vi "NotchFilter.vi"(3 "Image In":T1 {"Dialogs" format="%.0b"}) -> (0 "FFT Out":T1 {"Dialogs" format="%.0b"}, 1 "Image Out":T1 {"Dialogs" format="%.0b"})   [LabVIEW 2024]
doc: "This VI removes the mean (0 freq) from the image. It only works on greyscale images."
uses:
  <userlib>/ImageProcessing/QTLIB_2595_LV86/QT_Image.ctl
panel:
  # "This VI removes the mean (0 freq) from the image.  It only works on greyscale images."
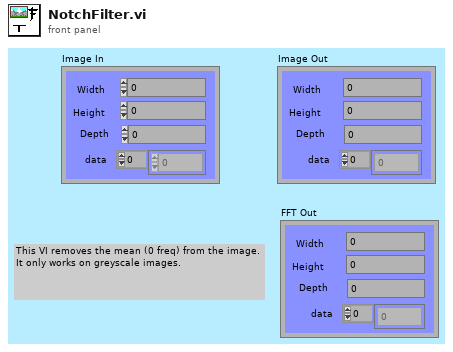
[diagram p1: front panel]
types:
  T1 = typedef "QT_Image.ctl" = cluster{"Width":i32, "Height":i32, "Depth":i32, "data":u8[], "Compressed data":u8[], "Color table":u32[], "Duration":i32, "Options":i32, "Timestamp":i32, "ID":i32, "Reserved":i32, "Dialogs":u32}
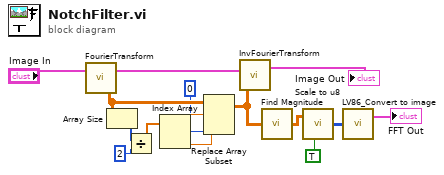
[diagram p0: block diagram]
diagram:
  n1 = call <userlib>:"FourierTransform.vi"("Image In"="Image In") -> ("Complex FT"=w15:cdb[][], "Image Out"=w5:T1)  [unwired: 1 in]
  n2 = Array Size(array=w15) -> (size(s)=w14:i32[])
  n3 = Divide(x=w14, y=2) -> (x/y=w12:dbl[])
  n4 = Index Array(array=w12) -> (element #1=w11:dbl, element #2=w10:dbl)  [unwired: 2 in]
  n5 = Replace Array Subset(array=w15, new element=0, index (row)=w11, index (col)=w10) -> (w3:cdb[][])
  n6 = call <userlib>:"InvFourierTransform.vi"("Complex matrix"=w3, "Image In"=w5) -> ("Image Out"=→"Image Out":T1)  [unwired: 1 in]
  n7 = call <userlib>:"Find Magnitude.vi"("FFT {X}"=w3) -> ("Magnitude"=w4:dbl[][])
  n8 = call <userlib>:"Scale to u8.vi"("Log scaling?"=TRUE, "Intensity Graph"=w4) -> ("X"=w6:u8[][])
  n9 = call <userlib>:"LV86_Convert to image.vi"("Intensity Graph"=w6) -> ("Image Out"=→"FFT Out":T1)  [unwired: 2 in]
